vi "fast_display_subVI_without_fileIO.vi"(9 "time informations":T1 {"length" format="%<%H:%M:%S%3u>t"}, 10 "acc waveform array":waveform(dbl)[](array[waveform]), 11 "input cluster":T3={"path to binary file"=path "C:/Users/Lenovo/Desktop/szakdoga/data", "Start Cursor"=timestamp(0 s since 1904-01-01), "Sec"=60.0, "crossing level"=-0.01, "threshold"=0.29999999999999993, "avg window size"=5, "peak detect width"=30, "invert"=FALSE, "SNR window width [Hz]"=0.5, "felharmonikus N"=2, "End cursor"=timestamp(0 s since 1904-01-01)} {"peak detect width" min=3; "threshold" format="%0.2f"}) -> (3 "data cluster":T2)   [LabVIEW 2017]
uses:
  LV Code/Controls/control_time_informations.ctl
  <vilib>/Analysis/1siggen.llb/Ramp Pattern by Samples.vi
  <vilib>/Analysis/1siggen.llb/Ramp Pattern by Delta.vi
  <vilib>/Waveform/WDTOps.llb/WDT Get Waveform Subset DBL.vi
  <vilib>/Analysis/NI_AALBase.lvlib
panel:
  in  "average window size":i32=5
  in  "low cutoff freq":dbl=0.05 format="%#_13g"
  in  "high cutoff freq":dbl=10.0 format="%#_13g"
  out "Z axis SNR":cluster{"Ramp Pattern":dbl[], dbl[]}[](graph)
  out "Y axis SNR":cluster{"Ramp Pattern":dbl[], dbl[]}[](graph)
  out "X axis SNR":cluster{"Ramp Pattern":dbl[], dbl[]}[](graph)
  out "resultant SNR":cluster{"Ramp Pattern":dbl[], dbl[]}[](graph)
  out "SNR":dbl
  out "csapás impulzus":cluster{"Ramp Pattern":dbl[], dbl[]}(graph)
  out "csapásszám":cluster{"Ramp Pattern":dbl[], dbl[]}[](graph)
  in  "felbontás [s]":dbl=20.0
  out "freq [Hz]":dbl
  out "PSD":cluster{"f0":dbl, "df":dbl, "magnitude":dbl[]}[](graph)
  out "inspection":cluster{"Y":dbl[], "Y":dbl[]}[](graph)
  out "inspected section":waveform(dbl)[](graph)
  out "read in data":waveform(dbl)[](graph)
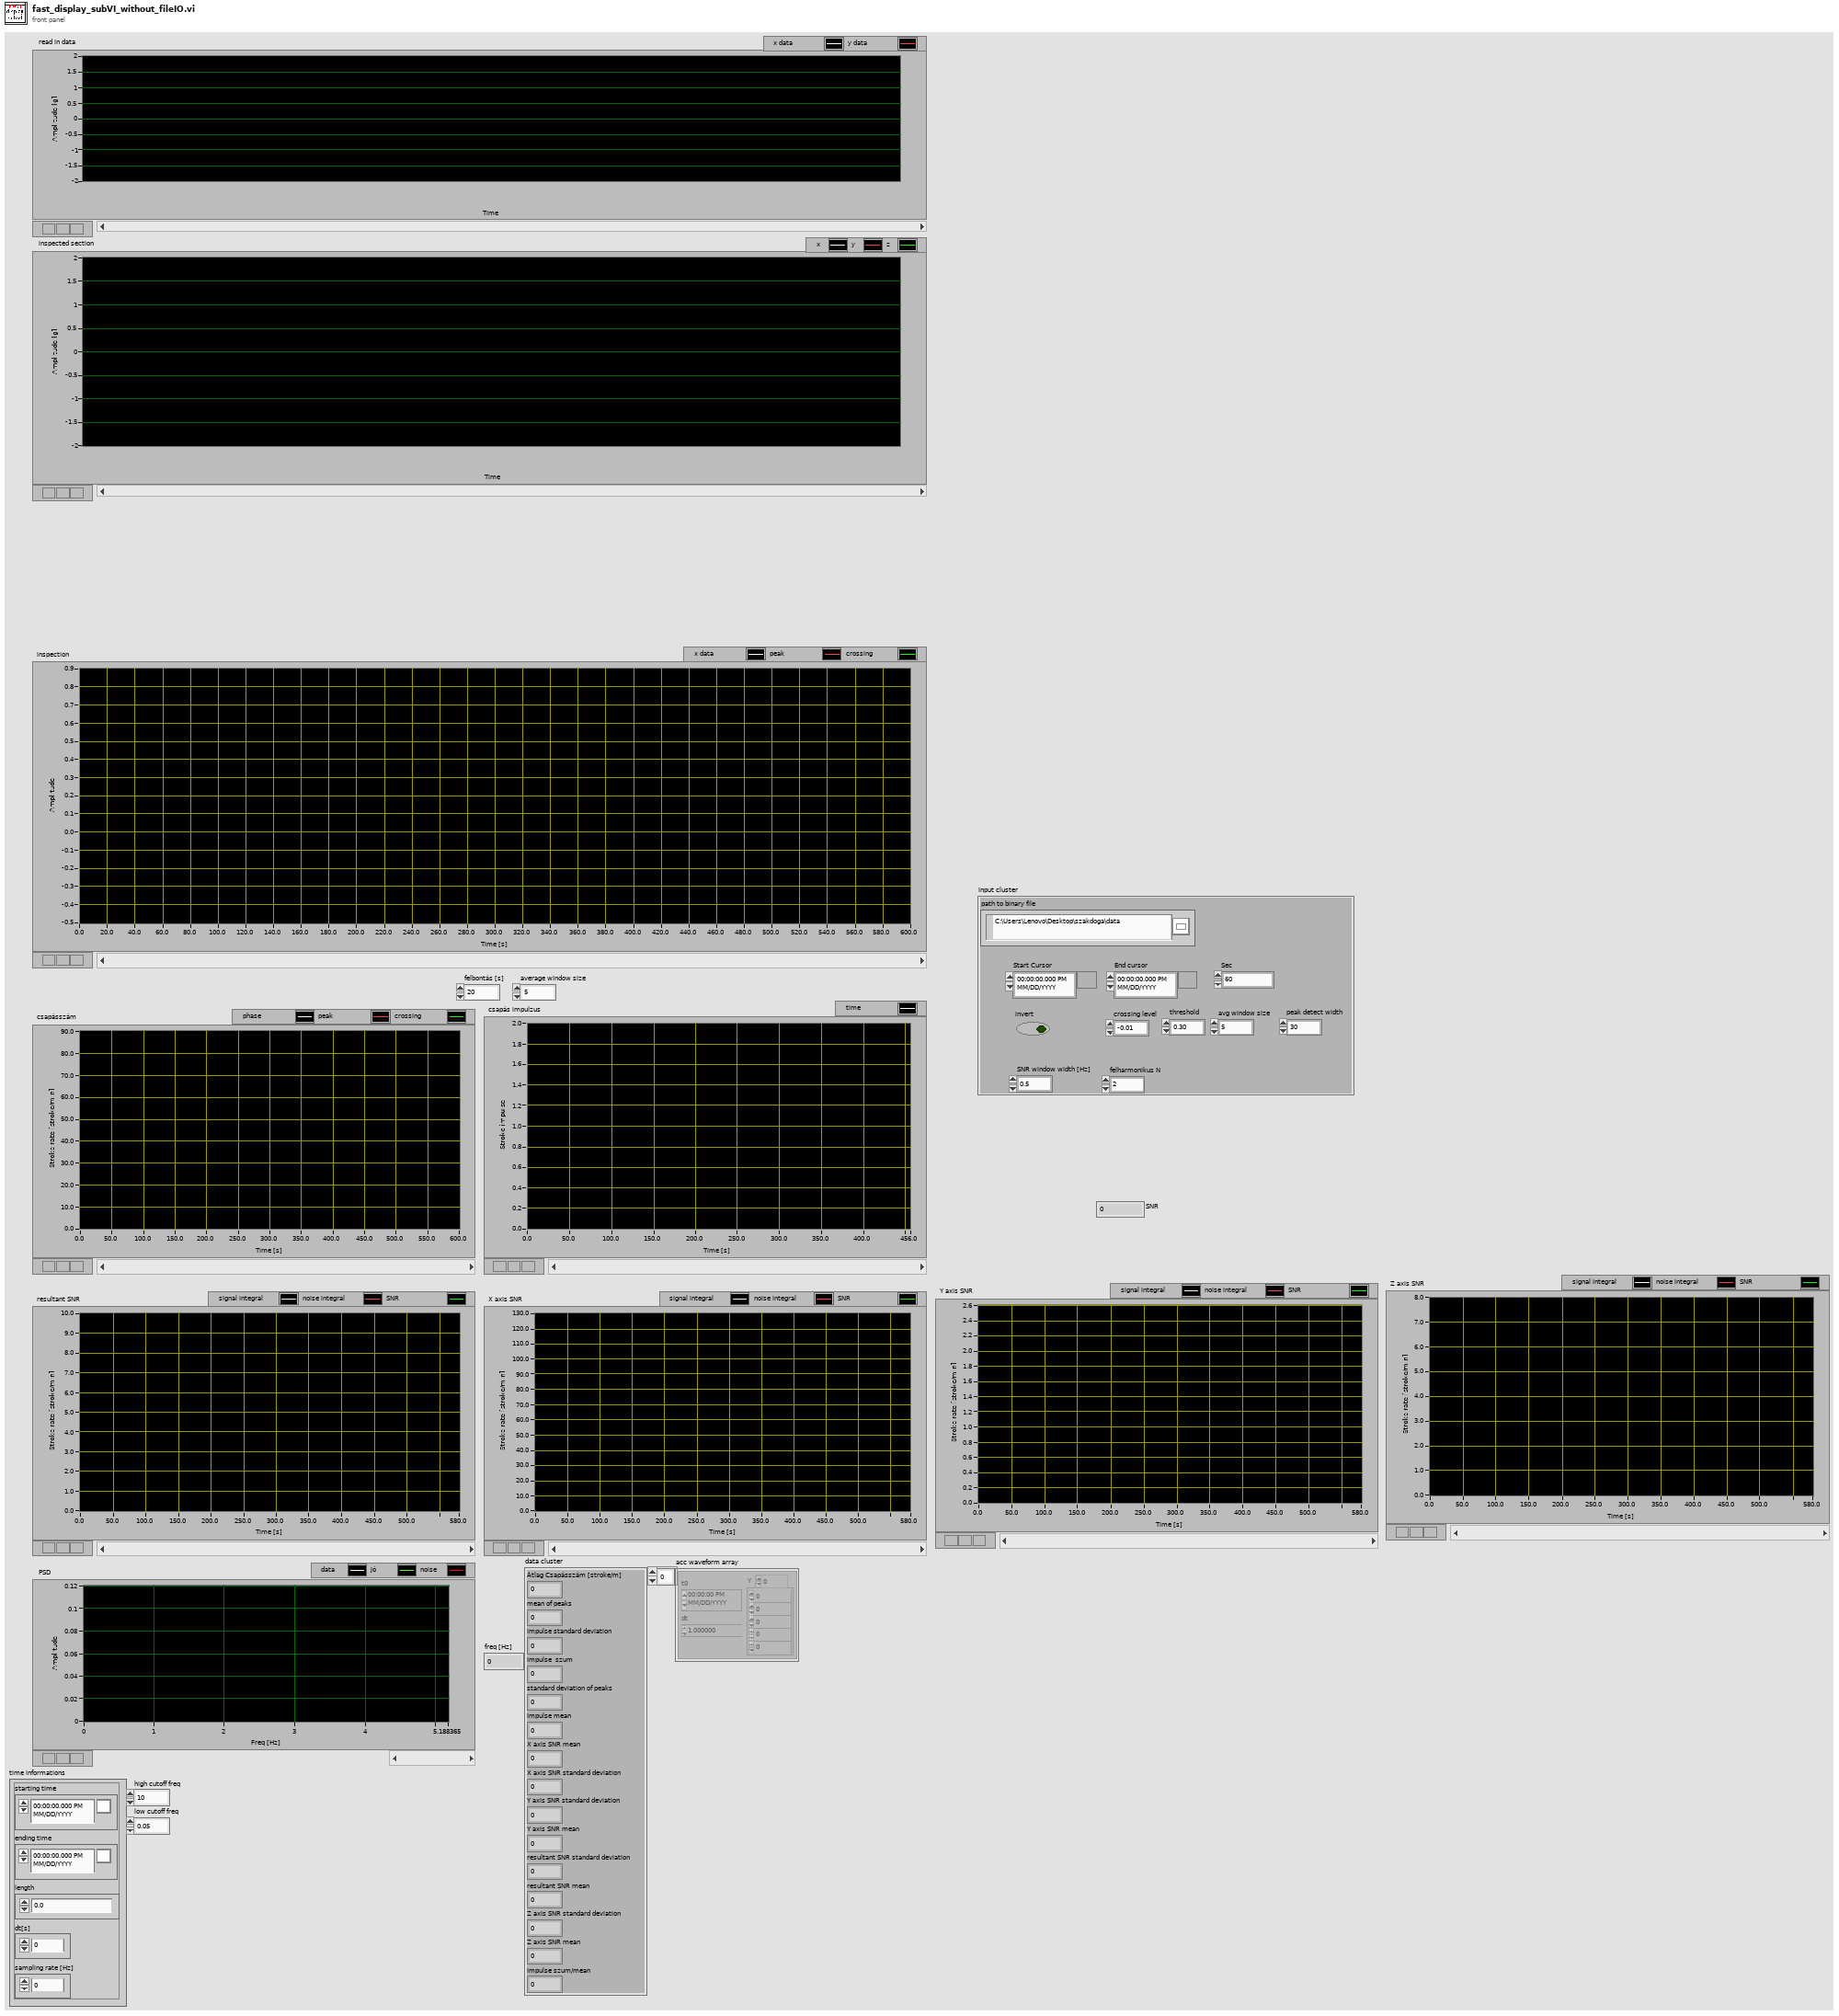
[diagram p1: front panel]
types:
  T1 = typedef "control_time_informations.ctl" = cluster{"starting time":timestamp, "ending time":timestamp, "dt[s]":dbl, "sampling rate [Hz]":dbl, "length":dbl}
  T2 = cluster{"Átlag Csapásszám [stroke/m]":dbl, "mean of peaks":dbl, "impulse standard deviation":dbl, "impulse  szum":dbl, "standard deviation of peaks":dbl, "impulse mean":dbl, "X axis SNR mean":dbl, "X axis SNR standard deviation":dbl, "Y axis SNR standard deviation":dbl, "Y axis SNR mean":dbl, "resultant SNR standard deviation":dbl, "resultant SNR mean":dbl, "Z axis SNR standard deviation":dbl, "Z axis SNR mean":dbl, "impulse szum/mean":dbl}
  T3 = cluster{"path to binary file":path, "Start Cursor":timestamp, "Sec":dbl, "crossing level":dbl, "threshold":dbl, "avg window size":i32, "peak detect width":i32, "invert":bool, "SNR window width [Hz]":dbl, "felharmonikus N":i32, "End cursor":timestamp}
  T4 = cluster{"Ramp Pattern":dbl[], "stroke rate":dbl[]}
  T5 = cluster{"Ramp Pattern":dbl[], "stroke rate":dbl[]}[]
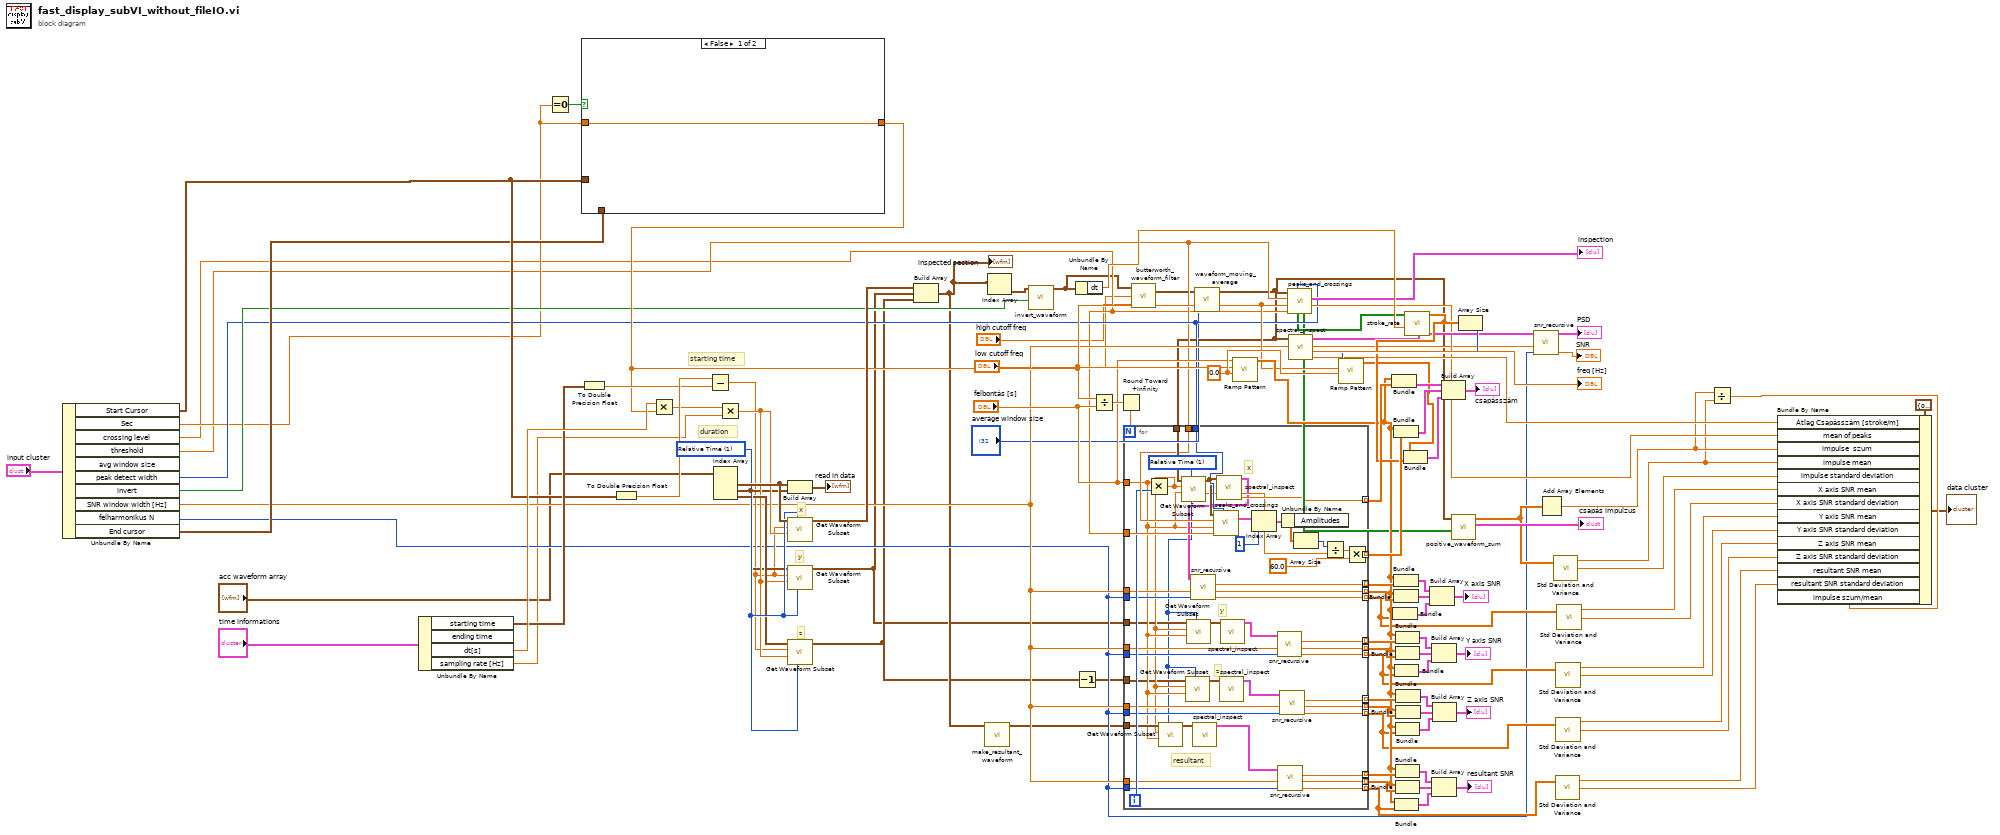
[diagram p0: block diagram]
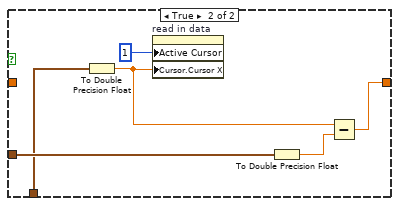
[diagram p2: hidden frame]
diagram:
  w85 = 0.0 ("start")
  w104 = u16 1 items=["Samples", "Relative Time"] ("start/duration format")
  # "duration"
  # "starting time"
  # "z"
  # "y"
  # "x"
  n1 = Unbundle By Name("input cluster") -> ("Start Cursor"=w30:timestamp, "Sec"=w24:dbl, "crossing level"=w20:dbl, "threshold"=w23:dbl, "peak detect width"=w25:i32, "invert"=w28:bool, "SNR window width [Hz]"=w27:dbl, "felharmonikus N"=w26:i32, "End cursor"=w29:timestamp)  [unwired: 1 out]
  n2 = Unbundle By Name("time informations") -> ("starting time"=w107:timestamp, "dt[s]"=w108:dbl, "sampling rate [Hz]"=w13:dbl)  [unwired: 1 out]
  n3 = Equal To 0?(x=w24) -> (x = 0?=w49:bool)
  n4 = case shown="False" w49 {
    tunnel: [w109 w113] -> w48
    tunnel: w24 -> [w109 _]
    tunnel: w30 -> [_ w112]
    tunnel: w29 -> [_ w111]
    frame False {
    }
    frame True {
      n5 = To Double Precision Float(number=w111) -> (double precision float=w110:dbl)
      n6 = property on="read in data" class="WFGraph (strict)"("Active Cursor"=1, "Cursor.Cursor X"=w110) -> ()  [unwired: 2 in, 2 out]
      n7 = To Double Precision Float(number=w112) -> (double precision float=w114:dbl)
      n8 = Subtract(x=w110, y=w114) -> (x-y=w113:dbl)
    }
  }
  n9 = To Double Precision Float(number=w107) -> (double precision float=w99:dbl)
  n10 = To Double Precision Float(number=w30) -> (double precision float=w100:dbl)
  n11 = Multiply(x=w108, y=w48) -> (x*y=w14:dbl)
  n12 = Subtract(x=w100, y=w99) -> (x-y=w98:dbl)
  n13 = Index Array(array="acc waveform array") -> (element #1=w105:waveform(dbl), element #2=w101:waveform(dbl), element #3=w103:waveform(dbl))  [unwired: 3 in]
  n14 = Multiply(x=w14, y=w13) -> (x*y=w102:dbl)
  n15 = Build Array(w105, w101) -> (→"read in data":waveform(dbl)[])
  n16 = call-poly <vilib>:"Get Waveform Subset.vi"("start/duration format"=w104, "duration"=w102, "start samples/time"=w98, "waveform in"=w105) -> ("waveform out"=w97:waveform(dbl))  [unwired: 2 in, 3 out]
  n17 = call-poly <vilib>:"Get Waveform Subset.vi"("start/duration format"=w104, "duration"=w102, "start samples/time"=w98, "waveform in"=w101) -> ("waveform out"=w15:waveform(dbl))  [unwired: 2 in, 3 out]
  n18 = call-poly <vilib>:"Get Waveform Subset.vi"("start/duration format"=w104, "duration"=w102, "start samples/time"=w98, "waveform in"=w103) -> ("waveform out"=w16:waveform(dbl))  [unwired: 2 in, 3 out]
  n19 = Build Array(w97, w15, w16) -> (w18:waveform(dbl)[])
  "inspected section" <- w18
  n20 = call "make_resultant_waveform.vi"("waveform array"=w18) -> ("inspected resultant"=w19:waveform(dbl))  [unwired: 10 in]
  n21 = Index Array(array=w18) -> (element=w88:waveform(dbl))  [unwired: 1 in]
  n22 = call "invert_waveform.vi"("invert"=w28, "waveform"=w88) -> ("output waveform"=w6:waveform(dbl))  [unwired: 9 in]
  n23 = Unbundle By Name(w6) -> ("dt"=w86:dbl)
  n24 = Decrement(x=w16) -> (x-1=w17:waveform(dbl))
  n25 = Divide(x=w48, y="felbontás [s]") -> (x/y=w94:dbl)
  n26 = Round Toward +Infinity(x=w94) -> (ceil(x): smallest int >= x=w95:dbl)
  n27 = call "butterworth_waveform_filter.vi"("high cutoff freq"="high cutoff freq", "low cutoff freq"="low cutoff freq", "input"=w6) -> ("filtered"=w3:waveform(dbl))  [unwired: 1 in]
  n28 = call "waveform_moving_average.vi"("window size"="average window size", "waveform"=w3) -> ("averaged waveform"=w2:waveform(dbl))  [unwired: 9 in]
  n29 = for {
    N: w95 -> [_]
    tunnel: "felbontás [s]" -> [w120]
    tunnel: w2 -> [w164]
    tunnel: [w163] -> w90 mode=indexing
    tunnel: [w155] -> w89 mode=indexing
    tunnel: w20 -> [w154]
    tunnel: w25 -> [w153]
    tunnel: w23 -> [w152]
    tunnel: w27 -> [w148]
    tunnel: w26 -> [w147]
    tunnel: [w146] -> w78 mode=indexing
    tunnel: [w145] -> w77 mode=indexing
    tunnel: [w144] -> w50 mode=indexing
    tunnel: w27 -> [w140]
    tunnel: w26 -> [w141]
    tunnel: [w138] -> w67 mode=indexing
    tunnel: [w142] -> w68 mode=indexing
    tunnel: [w143] -> w53 mode=indexing
    tunnel: w19 -> [w136]
    tunnel: w27 -> [w133]
    tunnel: w26 -> [w132]
    tunnel: [w134] -> w66 mode=indexing
    tunnel: [w131] -> w65 mode=indexing
    tunnel: [w130] -> w52 mode=indexing
    tunnel: w27 -> [w126]
    tunnel: w26 -> [w127]
    tunnel: [w125] -> w55 mode=indexing
    tunnel: [w128] -> w56 mode=indexing
    tunnel: [w129] -> w51 mode=indexing
    tunnel: w15 -> [w118]
    tunnel: w17 -> [w117]
    i -> [w150]
    w116 = u16 1 items=["Samples", "Relative Time"] ("start/duration format")
    # "resultant"
    # "z"
    # "y"
    # "x"
    n30 = Multiply(x=w120, y=w150) -> (x*y=w119:dbl)
    n31 = call-poly <vilib>:"Get Waveform Subset.vi"("start/duration format"=w116, "duration"=w120, "start samples/time"=w119, "waveform in"=w136) -> ("waveform out"=w137:waveform(dbl))  [unwired: 2 in, 3 out]
    n32 = call-poly <vilib>:"Get Waveform Subset.vi"("start/duration format"=w116, "duration"=w120, "start samples/time"=w119, "waveform in"=w164) -> ("actual duration"=w149:dbl, "waveform out"=w151:waveform(dbl))  [unwired: 2 in, 2 out]
    n33 = call-poly <vilib>:"Get Waveform Subset.vi"("start/duration format"=w116, "duration"=w120, "start samples/time"=w119, "waveform in"=w117) -> ("waveform out"=w124:waveform(dbl))  [unwired: 2 in, 3 out]
    n34 = call-poly <vilib>:"Get Waveform Subset.vi"("start/duration format"=w116, "duration"=w120, "start samples/time"=w119, "waveform in"=w118) -> ("waveform out"=w122:waveform(dbl))  [unwired: 2 in, 3 out]
    n35 = call "spectral_inspect.vi"("waveform"=w137) -> ("PSD"=w135:cluster{"f0":dbl, "df":dbl, "magnitude":dbl[]})  [unwired: 7 in, 3 out]
    n36 = call "peaks_and_crossings.vi"("width"=w153, "crossing level"=w154, "end"=w120, "threshold"=w152, "waveform"=w151) -> ("all in array"=w162:cluster{dbl[], "Amplitudes":dbl[]}[])  [unwired: 6 out]
    n37 = call "spectral_inspect.vi"("waveform"=w151) -> ("Csapásszám [stroke/min]"=w163:dbl, "PSD"=w139:cluster{"f0":dbl, "df":dbl, "magnitude":dbl[]})  [unwired: 7 in, 2 out]
    n38 = call "snr_recursive.vi"("felharmonikus N"=w141, "width [Hz]"=w140, "PSD"=w139) -> ("SNR"=w143:dbl, "Noise Integral"=w142:dbl, "Signal Integral"=w138:dbl)  [unwired: 5 in, 1 out]
    n39 = call "spectral_inspect.vi"("waveform"=w124) -> ("PSD"=w123:cluster{"f0":dbl, "df":dbl, "magnitude":dbl[]})  [unwired: 7 in, 3 out]
    n40 = call "spectral_inspect.vi"("waveform"=w122) -> ("PSD"=w121:cluster{"f0":dbl, "df":dbl, "magnitude":dbl[]})  [unwired: 7 in, 3 out]
    n41 = Index Array(array=w162, index=1) -> (element=w160:cluster{dbl[], "Amplitudes":dbl[]})
    n42 = call "snr_recursive.vi"("felharmonikus N"=w132, "width [Hz]"=w133, "PSD"=w121) -> ("SNR"=w130:dbl, "Noise Integral"=w131:dbl, "Signal Integral"=w134:dbl)  [unwired: 5 in, 1 out]
    n43 = call "snr_recursive.vi"("felharmonikus N"=w147, "width [Hz]"=w148, "PSD"=w135) -> ("SNR"=w144:dbl, "Noise Integral"=w145:dbl, "Signal Integral"=w146:dbl)  [unwired: 5 in, 1 out]
    n44 = call "snr_recursive.vi"("felharmonikus N"=w127, "width [Hz]"=w126, "PSD"=w123) -> ("SNR"=w129:dbl, "Noise Integral"=w128:dbl, "Signal Integral"=w125:dbl)  [unwired: 5 in, 1 out]
    n45 = Unbundle By Name(w160) -> ("Amplitudes"=w159:dbl[])
    n46 = Array Size(array=w159) -> (size(s)=w158:i32)
    n47 = Divide(x=w158, y=w149) -> (x/y=w157:dbl)
    n48 = Multiply(x=w157, y=60.0) -> (x*y=w155:dbl)
  }
  n49 = call-poly <vilib>:"Ramp Pattern.vi"("start"=w85, "end"=w48, "delta"="felbontás [s]") -> ("Ramp Pattern"=w54:dbl[])  [unwired: 6 in, 2 out]
  n50 = call "peaks_and_crossings.vi"("width"=w25, "crossing level"=w20, "end"=w48, "threshold"=w23, "waveform"=w2) -> ("mean of peaks"=w43:dbl, "all in array"=→"inspection":cluster{dbl[], "Amplitudes":dbl[]}[], "plus-minus"=w21:bool[], "minus-plus"=w22:bool[])  [unwired: 3 out]
  n51 = call "spectral_inspect.vi"("waveform"=w2) -> ("Csapásszám [stroke/min]"=w44:dbl, "freq"=→"freq [Hz]":dbl, "PSD"=w79:cluster{"f0":dbl, "df":dbl, "magnitude":dbl[]})  [unwired: 7 in, 1 out]
  n52 = Bundle("Ramp Pattern"=w54, w90) -> (w93:cluster{"Ramp Pattern":dbl[], dbl[]})  [unwired: 1 in]
  n53 = Bundle("Ramp Pattern"=w54, w53) -> (w71:cluster{"Ramp Pattern":dbl[], dbl[]})  [unwired: 1 in]
  n54 = Bundle("Ramp Pattern"=w54, w89) -> (w92:cluster{"Ramp Pattern":dbl[], dbl[]})  [unwired: 1 in]
  n55 = Bundle("Ramp Pattern"=w54, w67) -> (w69:cluster{"Ramp Pattern":dbl[], dbl[]})  [unwired: 1 in]
  n56 = Bundle("Ramp Pattern"=w54, w68) -> (w70:cluster{"Ramp Pattern":dbl[], dbl[]})  [unwired: 1 in]
  n57 = Bundle("Ramp Pattern"=w54, w52) -> (w62:cluster{"Ramp Pattern":dbl[], dbl[]})  [unwired: 1 in]
  n58 = Bundle("Ramp Pattern"=w54, w50) -> (w74:cluster{"Ramp Pattern":dbl[], dbl[]})  [unwired: 1 in]
  n59 = Bundle("Ramp Pattern"=w54, w66) -> (w64:cluster{"Ramp Pattern":dbl[], dbl[]})  [unwired: 1 in]
  n60 = Bundle("Ramp Pattern"=w54, w65) -> (w63:cluster{"Ramp Pattern":dbl[], dbl[]})  [unwired: 1 in]
  n61 = Bundle("Ramp Pattern"=w54, w51) -> (w59:cluster{"Ramp Pattern":dbl[], dbl[]})  [unwired: 1 in]
  n62 = Bundle("Ramp Pattern"=w54, w78) -> (w76:cluster{"Ramp Pattern":dbl[], dbl[]})  [unwired: 1 in]
  n63 = Bundle("Ramp Pattern"=w54, w77) -> (w75:cluster{"Ramp Pattern":dbl[], dbl[]})  [unwired: 1 in]
  n64 = Bundle("Ramp Pattern"=w54, w55) -> (w57:cluster{"Ramp Pattern":dbl[], dbl[]})  [unwired: 1 in]
  n65 = Bundle("Ramp Pattern"=w54, w56) -> (w58:cluster{"Ramp Pattern":dbl[], dbl[]})  [unwired: 1 in]
  n66 = call "stroke_rate.vi"("dt"=w86, "minus-plus"=w22) -> ("stroke rate"=w83:dbl[])  [unwired: 9 in]
  n67 = Build Array(w69, w70, w71) -> (→"X axis SNR":cluster{"Ramp Pattern":dbl[], dbl[]}[])
  n68 = Build Array(w64, w63, w62) -> (→"Y axis SNR":cluster{"Ramp Pattern":dbl[], dbl[]}[])
  n69 = Build Array(w76, w75, w74) -> (→"resultant SNR":cluster{"Ramp Pattern":dbl[], dbl[]}[])
  n70 = Build Array(w57, w58, w59) -> (→"Z axis SNR":cluster{"Ramp Pattern":dbl[], dbl[]}[])
  n71 = call "positive_waveform_sum.vi"("plus-minus"=w21, "waveform"=w2) -> ("csapás impulzus"=→"csapás impulzus":cluster{"Ramp Pattern":dbl[], dbl[]}, "Integral X"=w80:dbl[])  [unwired: 8 in]
  n72 = Array Size(array=w83) -> (size(s)=w84:i32)
  n73 = call-poly <vilib>:"Ramp Pattern.vi"("start"=w85, "end"=w48, "samples"=w84) -> ("Ramp Pattern"=w81:dbl[])  [unwired: 7 in, 1 out]
  n74 = Bundle("Ramp Pattern"=w81, "stroke rate"=w83) -> (w87:T4)  [unwired: 1 in]
  n75 = Build Array(w93, w92, w87) -> (→"csapásszám":T5)
  n76 = call "snr_recursive.vi"("felharmonikus N"=w26, "width [Hz]"=w27, "PSD"=w79) -> ("SNR"=→"SNR":dbl, "PSD"=→"PSD":cluster{"f0":dbl, "df":dbl, "magnitude":dbl[]}[])  [unwired: 5 in, 2 out]
  n77 = Add Array Elements(numeric array=w80) -> (sum=w12:dbl)
  n78 = call <vilib>:"Std Deviation and Variance.vi"("X"=w80) -> ("mean"=w11:dbl, "standard deviation"=w42:dbl)  [unwired: 1 in, 1 out]
  n79 = call <vilib>:"Std Deviation and Variance.vi"("X"=w50) -> ("mean"=w35:dbl, "standard deviation"=w34:dbl)  [unwired: 1 in, 1 out]
  n80 = call <vilib>:"Std Deviation and Variance.vi"("X"=w52) -> ("mean"=w39:dbl, "standard deviation"=w38:dbl)  [unwired: 1 in, 1 out]
  n81 = call <vilib>:"Std Deviation and Variance.vi"("X"=w51) -> ("mean"=w37:dbl, "standard deviation"=w36:dbl)  [unwired: 1 in, 1 out]
  n82 = call <vilib>:"Std Deviation and Variance.vi"("X"=w53) -> ("mean"=w41:dbl, "standard deviation"=w40:dbl)  [unwired: 1 in, 1 out]
  n83 = Divide(x=w12, y=w11) -> (x/y=w10:dbl)
  n84 = Bundle By Name ("data")(cluster=T2 {"Átlag Csapásszám [stroke/m]"=0.0, "mean of peaks"=0.0, "impulse standard deviation"=0.0, "impulse  szum"=0.0, "standard deviation of peaks"=0.0, "impulse mean"=0.0, "X axis SNR mean"=0.0, "X axis SNR standard deviation"=0.0, "Y axis SNR standard deviation"=0.0, "Y axis SNR mean"=0.0, "resultant SNR standard deviation"=0.0, "resultant SNR mean"=0.0, "Z axis SNR standard deviation"=0.0, "Z axis SNR mean"=0.0, "impulse szum/mean"=0.0} ("input cluster"), "Átlag Csapásszám [stroke/m]"=w44, "mean of peaks"=w43, "impulse  szum"=w12, "impulse mean"=w11, "impulse standard deviation"=w42, "X axis SNR mean"=w41, "X axis SNR standard deviation"=w40, "Y axis SNR mean"=w39, "Y axis SNR standard deviation"=w38, "Z axis SNR mean"=w37, "Z axis SNR standard deviation"=w36, "resultant SNR mean"=w35, "resultant SNR standard deviation"=w34, "impulse szum/mean"=w10) -> (→"data cluster":T2)
